vi "Result.Build FileDataObject.vi"(7 "Catagory":string, 10 "Name":string, 11 "File":path) -> (3 "ResultObj":T1)   [LabVIEW 2018]
uses:
  Reports/Report.Result FileDataObject.ctl
  <vilib>/KATE/Files/File Utils.lvlib
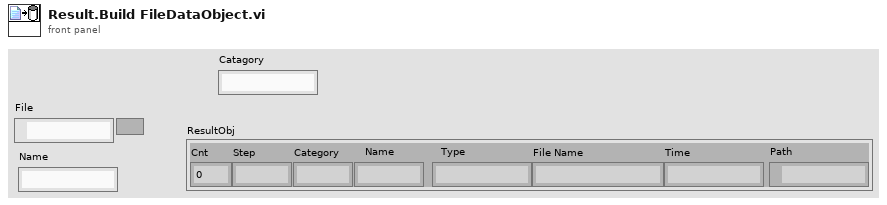
[diagram p1: front panel]
types:
  T1 = typedef "Report.Result FileDataObject.ctl" = cluster{"Cnt":i32, "Step":string, "Category":string, "Name":string, "Type":string, "File Name":string, "Time":string, "Path":path}
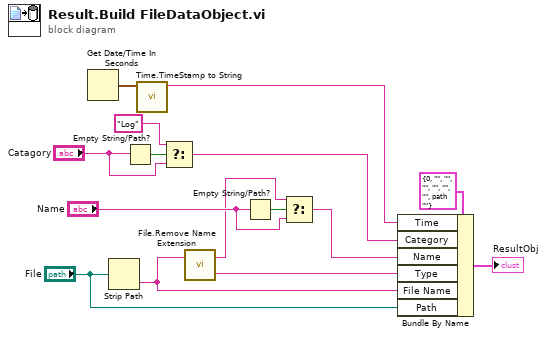
[diagram p0: block diagram]
diagram:
  n1 = Get Date/Time In Seconds() -> (seconds since 1Jan1904=w14:timestamp)
  n2 = Strip Path(path="File") -> (name=w10:string)  [unwired: 1 out]
  n3 = Empty String/Path?(string/path="Catagory") -> (empty?=w9:bool)
  n4 = call "Time.TimeStamp to String.vi"("Time Stamp in"=w14) -> ("Time String Out"=w13:string)  [unwired: 10 in]
  n5 = Select(t="Log" ("Category"), s=w9, f="Catagory") -> (s? t:f=w6:string)
  n6 = call <vilib>:"File.Remove Name Extension.vi"("File Name"=w10) -> ("Ext"=w12:string, "Name Less Ext"=w3:string)  [unwired: 1 in]
  n7 = Empty String/Path?(string/path="Name") -> (empty?=w5:bool)
  n8 = Select(t=w3, s=w5, f="Name") -> (s? t:f=w2:string)
  n9 = Bundle By Name(cluster=T1 {"Cnt"=0, "Step"="", "Category"="", "Name"="", "Type"="", "File Name"="", "Time"="", "Path"=path ""} ("FileData Object"), "Time"=w13, "Category"=w6, "Name"=w2, "Type"=w12, "File Name"=w10, "Path"="File") -> (→"ResultObj":T1)
